vi "get&set FileName.vi"(6 "Get/Set? (Set)":bool=TRUE, 8 "error in (no error)":errorcluster, 10 "FileName":path, 11 "VGS_VolumeDescriptor+File in":refnum<class "VGS_VolumeDescriptor+File.lvclass">) -> (0 "error out":errorcluster, 2 "FileName":path, 3 "VGS_VolumeDescriptor+File out":refnum<class "VGS_VolumeDescriptor+File.lvclass">)   [LabVIEW 2022 SP3, in "LV_VGS.lvlib" / "VGS_VolumeDescriptor+File.lvclass"]
doc: "<B>Defines physical position of a single slice file. </B>\n\nDefines the relative physical position of a single slice file. Use this function if the file represents a single xy-slice (z-size is 1).\n\nThis function is equivalent to calling setPositionList() with a list of size 1. See setPositionList() for details. \n\n<B>bool VGS::Project::Interop::VolumeDescriptor::File::setPositionList ( List< float >^ positionList ) </B>\n\nDefines physical positions of the file's slices. \n\nDefines the relative physical position of all the slices represented by this file. Use this function to define non-equidistant slices: normally, the slice distance is determined globally by the z-component of VolumeDescriptor.Resolution, i.e. all given xy-slices are the same distance apart. If your scanned data has varying slice distances, however, you can define a kind of physical position (in mm) for each slice. These distances will then be used instead of the z-resolution value, which will be ignored.\n\n You cannot \"mix\" specifications: if you specify a position list, you must do it for all files in the VolumeDescriptor, and each file must specify as many positions as its z-size indicates! \n Optional definition. The default value is an empty list."
uses:
  VGS_VolumeDescriptor+File.lvclass
  VGS_VolumeDescriptor+File.lvclass/VGS_VolumeDescriptor+File.ctl
  C:/Users/Andrey/Documents/GitHub/LV_VGS/vgs_project.dll
  vgs_project.dll
panel:
  # "-Set\n-Get"
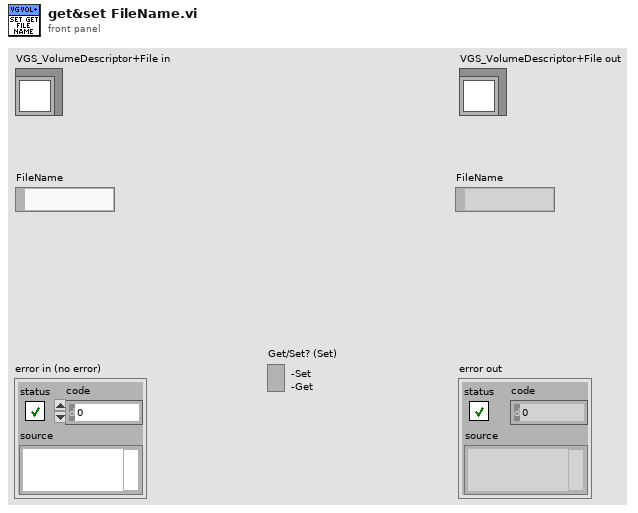
[diagram p1: front panel]
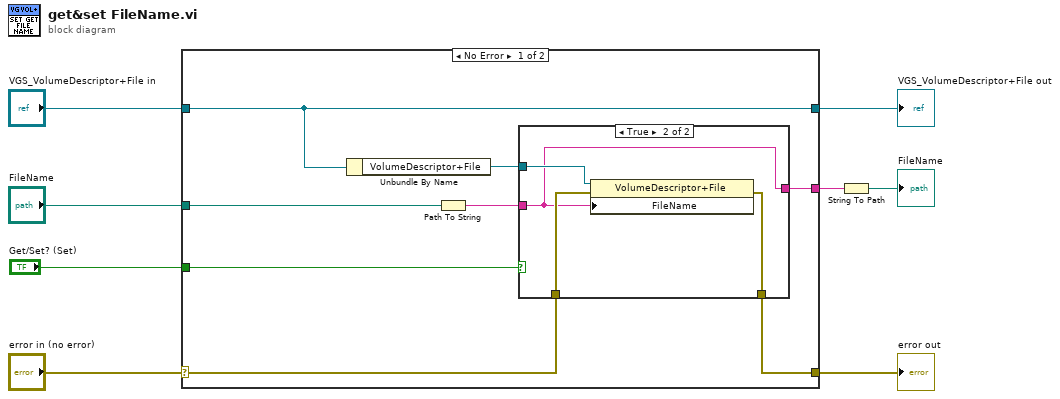
[diagram p0: block diagram]
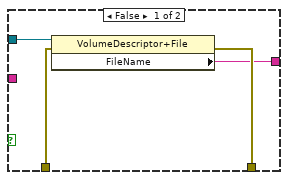
[diagram p2: hidden frame]
diagram:
  n1 = case shown="No Error" "error in (no error)" {
    selector: "error in (no error)" -> [w14 w26]
    tunnel: [w13 w26] -> w7
    tunnel: [w16 w25] -> w5
    tunnel: "VGS_VolumeDescriptor+File in" -> [w16 w25]
    tunnel: [w12 _] -> w4
    tunnel: "Get/Set? (Set)" -> [w11 _]
    tunnel: "FileName" -> [w10 _]
    frame No Error {
      n2 = Unbundle By Name(w16) -> ("VolumeDescriptor+File"=w15:refnum<k24>)
      n3 = Path To String(path=w10) -> (string=w9:string)
      n4 = case shown="True" w11 {
        tunnel: w15 -> [w20 w22]
        tunnel: w14 -> [w19 w24]
        tunnel: [w18 w23] -> w13
        tunnel: [w17 w21] -> w12
        tunnel: w9 -> [_ w21]
        frame False {
          n5 = property class="VolumeDescriptor+File"(reference=w20, error in=w19) -> (error out=w18:errorcluster, "FileName"=w17:string)  [unwired: 1 out]
        }
        frame True {
          n6 = property class="VolumeDescriptor+File"(reference=w22, error in=w24, "FileName"=w21) -> (error out=w23:errorcluster)  [unwired: 1 out]
        }
      }
    }
    frame Error {
    }
  }
  "error out" <- w7
  "VGS_VolumeDescriptor+File out" <- w5
  n7 = String To Path(string=w4) -> (path=→"FileName":path)
